vi "PrefsGlobal.vi"() -> ()   [LabVIEW 2013]
uses:
  SetListPrefs/SetListPrefs.lvclass
panel:
  in  "SetListPrefs.lvclass":refnum<class "SetListPrefs.lvclass">
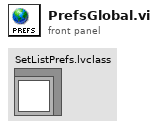
[diagram p1: front panel]
diagram:
